vi "配置文件全局.vi"() -> ()   [LabVIEW 2013]
panel:
  in  "供电电源偏差":dbl
  in  "供电电源基准":dbl
  in  "诊断标定读取地址":path=path "E:/"
  in  "参数生成器读取地址":path=path "E:/"
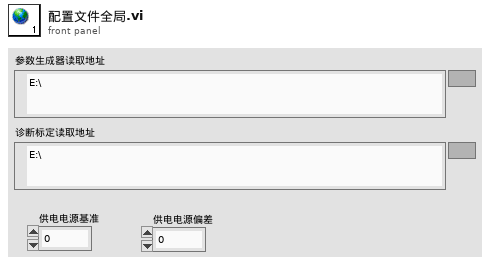
[diagram p1: front panel]
diagram:
